vi "Read Range.vi"(0 "VISA resource name":refnum<visa-resource-name>, 11 "error in (no error)":errorcluster) -> (4 "VISA resource name out":refnum<visa-resource-name>, 6 "Range":dbl format="%.2f", 15 "error out":errorcluster)   [LabVIEW 2014, in "Yokogawa.lvlib" / "Yokogawa PZ4000.lvlib"]
doc: "This VI reads the Range from the PZ4000 series.\nNOTE : Returns the Range value for the waveform designated by \"YKPZ4000 Config Waveform.vi (Select Trace)\"."
uses:
  Yokogawa PZ4000.lvlib
panel:
  # "NOTE : Returns the Range value for \nthe waveform designated by \n\"YKPZ4000 Config Waveform.vi \n(Select Trace)\"."
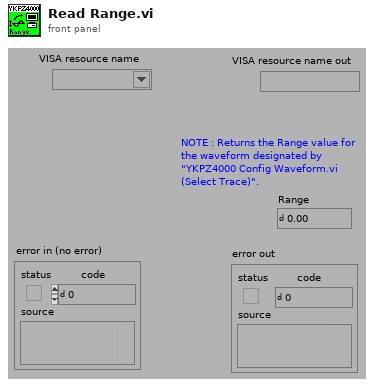
[diagram p1: front panel]
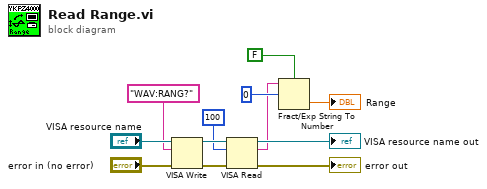
[diagram p0: block diagram]
diagram:
  n1 = VISA Write(VISA resource name="VISA resource name", write buffer="WAV:RANG?", error in (no error)="error in (no error)") -> (VISA resource name out=w6:refnum<visa-resource-name>, error out=w12:errorcluster)  [unwired: 1 out]
  n2 = VISA Read(VISA resource name=w6, byte count=100, error in (no error)=w12) -> (VISA resource name out=→"VISA resource name out":refnum<visa-resource-name>, read buffer=w2:string, error out=→"error out":errorcluster)  [unwired: 1 out]
  n3 = Fract/Exp String To Number(use system decimal point (T)=FALSE ("¼½ÃÑ10i¬_ðgp(T)"), string=w2, offset=0) -> (number=→"Range":dbl)  [unwired: 1 in, 1 out]
